vi "ics_ids_save_2D_2ch.vi"(0 "pixels 2":i32, 1 "filename 2":string, 3 "folder 2":path=path "D:/User/Sergey/ids_ics_trainer", 5 "Dwell 2":dbl, 7 "data":i32[][](array[numeric]), 9 "Range 2":dbl, 11 "error in":errorcluster, 12 "data 2":dbl[][](array[numeric])) -> (4 "saved":bool, 15 "error out":errorcluster)   [LabVIEW 2016]
panel:
  in  "scale I 2":i32=1
  out "path to .ids":path
  out "saved 2":bool
  out "text 2":string
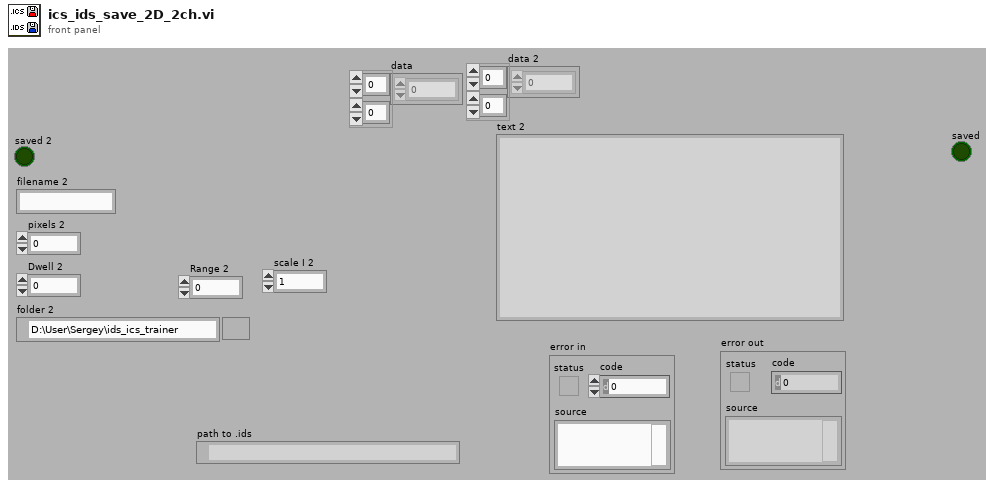
[diagram p1: front panel]
types:
  T1 = enum16{"open", "replace", "create", "open or create", "replace or create", "replace or create with confirmation"}
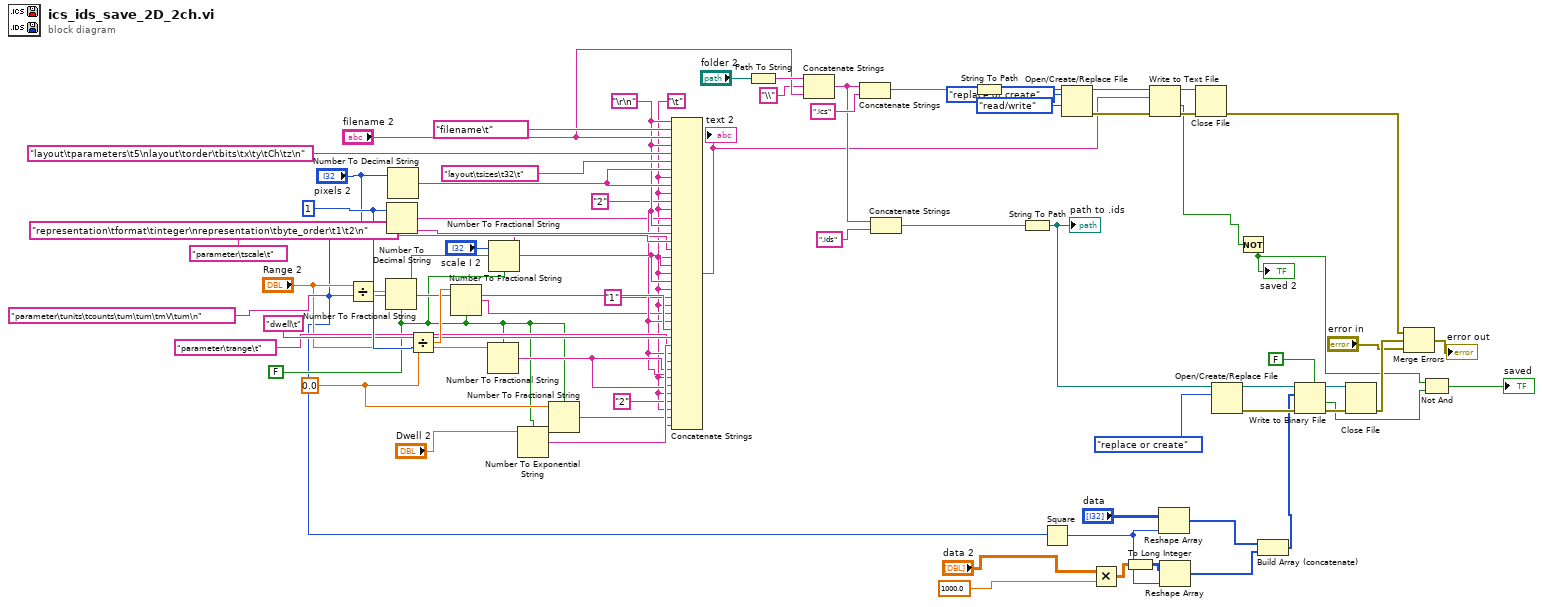
[diagram p0: block diagram]
diagram:
  w35 = 1 ("slices Z")
  w26 = 0.0 ("Range Z")
  w23 = FALSE ("use system decimal point (T)")
  w13 = "\t"
  w22 = "\r\n"
  n1 = Divide(x="Range 2", y="pixels 2") -> (x/y=w39:dbl)
  n2 = Number To Fractional String(use system decimal point (T)=w23, number=w39) -> (F-format string=w36:string)  [unwired: 2 in]
  n3 = Number To Decimal String(number=w35) -> (decimal integer string=w18:string)  [unwired: 1 in]
  n4 = Number To Decimal String(number="pixels 2") -> (decimal integer string=w42:string)  [unwired: 1 in]
  n5 = Divide(x=w26, y=w35) -> (x/y=w34:dbl)
  n6 = Number To Fractional String(use system decimal point (T)=w23, number=w34) -> (F-format string=w17:string)  [unwired: 2 in]
  n7 = Number To Fractional String(use system decimal point (T)=w23, number="Range 2") -> (F-format string=w27:string)  [unwired: 2 in]
  n8 = Number To Fractional String(use system decimal point (T)=w23, number="scale I 2") -> (F-format string=w37:string)  [unwired: 2 in]
  n9 = Number To Exponential String(number="Dwell 2", 1:w23) -> (E-format string=w30:string)  [unwired: 2 in]
  n10 = Number To Fractional String(use system decimal point (T)=w23, number=w26) -> (F-format string=w15:string)  [unwired: 2 in]
  n11 = Concatenate Strings(w22, "filename\t" ("string"), "filename 2", w22, "layout\tparameters\t5\nlayout\torder\tbits\tx\ty\tCh\tz\n" ("string"), "layout\tsizes\t32\t" ("string"), w42, w13, w42, w13, "2" ("string"), w13, w18, w22, "representation\tformat\tinteger\nrepresentation\tbyte_order\t1\t2\n" ("string"), "parameter\tscale\t" ("string"), w37, w13, w36, w13, w36, w13, "1" ("string"), w13, w17, w22, "parameter\tunits\tcounts\tum\tum\tmV\tum\n" ("string"), "dwell\t" ("string"), w30, w22, "parameter\trange\t" ("string"), w27, w13, w27, w13, "2" ("string"), w13, w15, w22) -> (w43:string)
  "text 2" <- w43
  n12 = Path To String(path="folder 2") -> (string=w52:string)
  n13 = Concatenate Strings(w52, "\\" ("string"), "filename 2") -> (w45:string)
  n14 = Concatenate Strings(w45, ".ics" ("string")) -> (w47:string)
  n15 = Concatenate Strings(w45, ".ids" ("string")) -> (w44:string)
  n16 = String To Path(string=w47) -> (path=w51:path)
  n17 = String To Path(string=w44) -> (path=w12:path)
  "path to .ids" <- w12
  n18 = Square(x="pixels 2") -> (x^2=w8:i32)
  n19 = Open/Create/Replace File(file path (use dialog)=w51, operation (0:open)=T1."replace or create", access (0:read/write)=enum16{"read/write", "read-only", "write-only"}."read/write") -> (refnum out=w54:refnum<file>, error out=w53:errorcluster)  [unwired: 3 in, 1 out]
  n20 = Multiply(x="data 2", y=1000.0) -> (x*y=w2:dbl[][])
  n21 = To Long Integer(number=w2) -> (32bit integer=w1:i32[][])
  n22 = Write to Text File(file (use dialog)=w54, text=w43, error in=w53) -> (refnum out=w56:refnum<file>, cancelled=w21:bool, error out=w55:errorcluster)  [unwired: 1 in]
  n23 = Reshape Array("data", w8) -> (w6:i32[])
  n24 = Reshape Array(w1, w8) -> (w4:i32[])
  n25 = Close File(refnum=w56, error in=w55) -> (error out=w10:errorcluster)  [unwired: 1 out]
  n26 = Open/Create/Replace File(file path (use dialog)=w12, operation (0:open)=T1."replace or create") -> (refnum out=w68:refnum<file>, error out=w67:errorcluster)  [unwired: 4 in, 1 out]
  n27 = Not(x=w21) -> (.not. x?=w11:bool)
  "saved 2" <- w11
  n28 = Build Array (concatenate)(w6, w4) -> (w5:i32[])
  n29 = Write to Binary File(file (use dialog)=w68, data=w5, error in=w67, 5:FALSE ("prepend array or string size? (T)")) -> (refnum out=w69:refnum<file>, cancelled=w62:bool, error out=w70:errorcluster)  [unwired: 2 in]
  n30 = Close File(refnum=w69, error in=w70) -> (error out=w65:errorcluster)  [unwired: 1 out]
  n31 = Merge Errors(w10, w65, "error in") -> (→"error out":errorcluster)
  n32 = Not And(1:w62, 2:w11) -> (0:→"saved":bool)
